vi "H036 Harsh Pandit SCADA Lab 6b Sem 6.vi"() -> ()   [LabVIEW 2018]
panel:
  out "Array 2":bool[](array[boolean])
  out "Rotated Array":dbl[](array[numeric])
  in  "Array":dbl[](array[numeric])
  # "Experiment 6b: Create 1 D numeric array which consist of 10 elements and rotate it 10 times.\nFor each rotation, display equivalent binary number of first array element in form of boolean\narray."
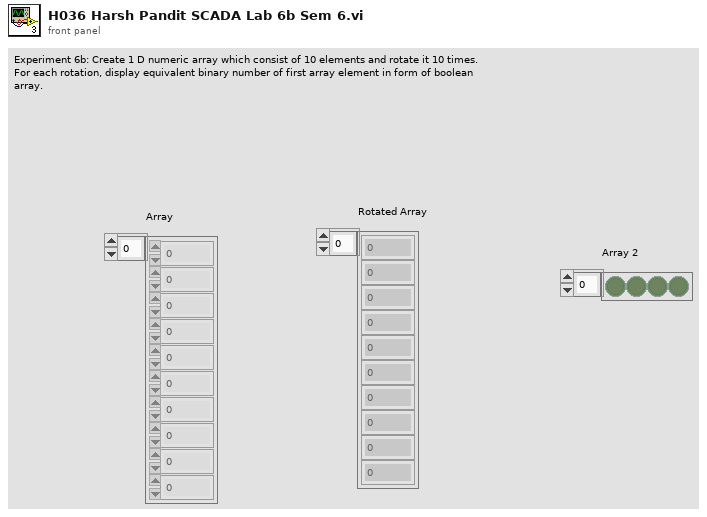
[diagram p1: front panel]
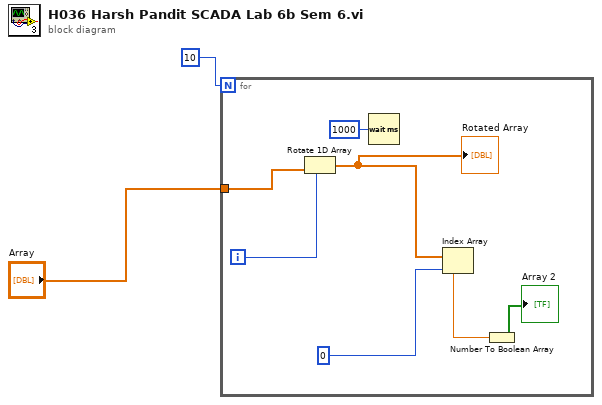
[diagram p0: block diagram]
diagram:
  n1 = for {
    N: 10 -> [_]
    tunnel: "Array" -> [w5]
    i -> [w8]
    n2 = Rotate 1D Array(1:w5, 2:w8) -> (0:w7:dbl[])
    "Rotated Array" <- w7
    n3 = Wait (ms)(milliseconds to wait=u32 1000) -> ()  [unwired: 1 out]
    n4 = Index Array(array=w7, index=0 ("index (row)")) -> (element=w4:dbl)
    n5 = Number To Boolean Array(number=w4) -> (Boolean array=→"Array 2":bool[])
  }
